vi "Condition Add.vi"(8 "error in (no error)":errorcluster, 9 "Condition":T2, 10 "ixScenario (0)":i32, 11 "Connection Refnum":T1) -> (0 "error out":errorcluster, 3 "Connection Refnum":T1)   [LabVIEW 2011]
uses:
  Condition Record.ctl
  Condition Operators.ctl
  SI.LIB/ODBC/SQL Controls/Connection Refnum.ctl
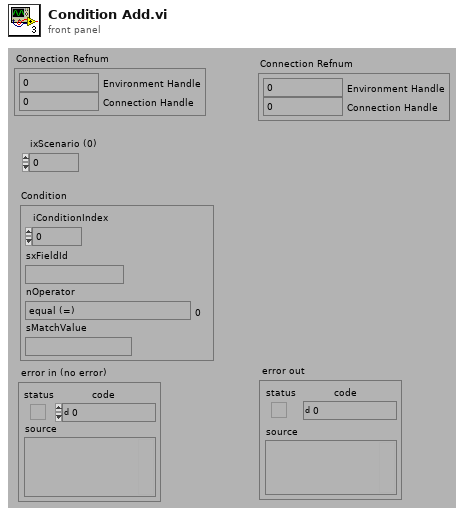
[diagram p1: front panel]
types:
  T1 = typedef "Connection Refnum.ctl" = cluster{"Environment Handle":i32, "Connection Handle":i32}
  T2 = typedef "Condition Record.ctl" = cluster{"iConditionIndex":i32, "sxFieldId":string, "nOperator":T3, "sMatchValue":string}
  T3 = typedef "Condition Operators.ctl" = enum16{"equal (=)", "not equal (\\u2260)", "less than (<)", "less than or equal (\\u2264)", "greater than (>)", "greater than or equal (\\u2265)", "contains", "does not contain"}
  T4 = typedef "Statement Refnum.ctl" = cluster{"Statement Handle":i32, "Parameter Number":u16}
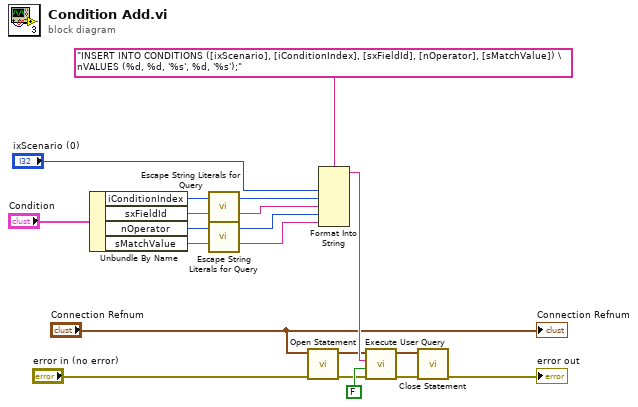
[diagram p0: block diagram]
diagram:
  n1 = Unbundle By Name("Condition") -> ("iConditionIndex"=w2:i32, "sxFieldId"=w11:string, "nOperator"=w1:T3, "sMatchValue"=w12:string)
  n2 = call "Escape String Literals for Query.vi"("String"=w11) -> ("escaped String"=w10:string)  [unwired: 1 in, 13 out]
  n3 = call "Escape String Literals for Query.vi"("String"=w12) -> ("escaped String"=w9:string)  [unwired: 1 in, 13 out]
  n4 = call "Open Statement.vi"("error in (no error)"="error in (no error)", "Connection Refnum"="Connection Refnum") -> ("error out"=w14:errorcluster, "Statement Refnum"=w13:T4)  [unwired: 4 out]
  n5 = Format Into String(format string="INSERT INTO CONDITIONS ([ixScenario], [iConditionIndex], [sxFieldId], [nOperator], [sMatchValue]) \nVALUES (%d, %d, '%s', %d, '%s');" ("User Query"), "ixScenario (0)", w2, w10, w1, w9) -> (resulting string=w18:string)  [unwired: 2 in, 1 out]
  n6 = call "Execute User Query.vi"("error in (no error)"=w14, "Return Data? (f)"=FALSE, "User Query"=w18, "Statement Refnum"=w13) -> ("error out"=w15:errorcluster, "Statement Refnum"=w16:T4)  [unwired: 2 out]
  n7 = call "Close Statement.vi"("error in (no error)"=w15, "Statement Refnum"=w16) -> ("error out"=→"error out":errorcluster)  [unwired: 5 out]
  "Connection Refnum" <- "Connection Refnum"
